vi "Start.vi"(8 "error in (no error)":errorcluster, 9 "Timing":T1, 11 "State in":refnum<class "State.lvclass">) -> (0 "error out":errorcluster, 3 "State out":refnum<class "State.lvclass">)   [LabVIEW 2020, in "VolatusSeq.lvlib" / "State.lvclass"]
uses:
  State.lvclass
  State.lvclass/State.ctl
  Timing.ctl
  VolatusSeq.lvlib
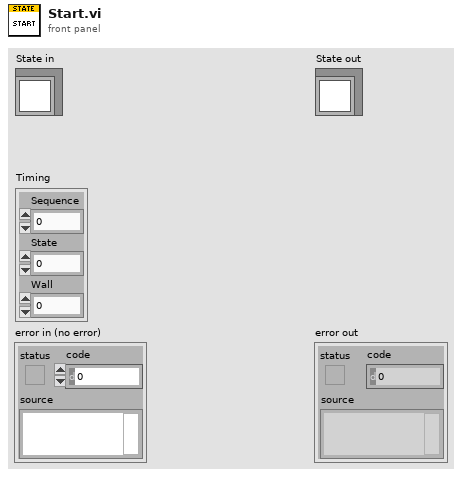
[diagram p1: front panel]
types:
  T1 = typedef "VolatusSeq.lvlib/Timing.ctl" = cluster{"Sequence":dbl, "State":dbl, "Wall":dbl}
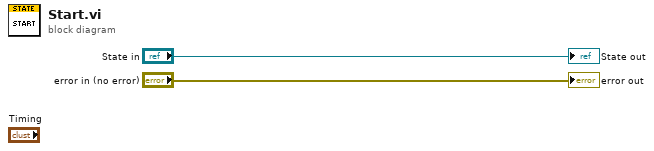
[diagram p0: block diagram]
diagram:
  "error out" <- "error in (no error)"
  "State out" <- "State in"
